vi "Estimate Ackermann Steering Frame.vi"(8 "error in (no error)":errorcluster, 11 "steering frame in":refnum<class "NI_Robotics_Steering Frame.lvclass">) -> (0 "error out":errorcluster, 2 "estimated ackermann steering frame copy":refnum<class "NI_Robotics_Ackermann Steering Frame.lvclass">, 3 "steering frame out":refnum<class "NI_Robotics_Steering Frame.lvclass">)   [LabVIEW 2017, in "NI_Robotics_Configure Steering Frame.lvlib"]
uses:
  <vilib>/robotics/Dialog/Configure Steering Frame/NI_Robotics_Configure Steering Frame.lvlib
  <vilib>/robotics/Steering/Steering Frame/NI_Robotics_Steering Frame.lvclass
  <vilib>/robotics/Steering/Ackermann Steering Frame/NI_Robotics_Ackermann Steering Frame.lvclass
  <vilib>/robotics/Steering/Steering Frame/NI_Robotics_Steering Frame.lvclass/NI_Robotics_Steering Frame.ctl
  <vilib>/robotics/Steering/Wheel/Wheel Parameters.ctl
  <vilib>/robotics/Steering/Wheel/Rotation Direction.ctl
  <vilib>/robotics/Steering/Steering Wheel/Steering Wheel Parameters.ctl
  <vilib>/robotics/Steering/Steering Wheel/Steering Angle Range.ctl
  <vilib>/robotics/Steering/Fixed Wheel/NI_Robotics_Fixed Wheel.lvclass
  c:/Program Files (x86)/National Instruments/LabVIEW 2017/vi.lib/robotics/Steering/Wheel/NI_Robotics_Wheel.lvclass
  <vilib>/robotics/Steering/Steering Wheel/NI_Robotics_Steering Wheel.lvclass
  <vilib>/robotics/Steering/Wheel/NI_Robotics_Wheel.lvclass/NI_Robotics_Wheel.ctl
  <vilib>/robotics/Steering/Steering Frame/Get Multiple Wheels in Steering Frame.vi
  <vilib>/robotics/Steering/Wheel/Get General Wheel Information.vi
  <vilib>/robotics/Steering/Wheel/Get Wheel Radius.vi
  <vilib>/robotics/Steering/Wheel/Get Motor Communication.vi
  <vilib>/robotics/Steering/Wheel/Get Wheel Parameters.vi
  <vilib>/robotics/Steering/Ackermann Steering Frame/Create Ackermann Steering Frame.vi
  <vilib>/robotics/Steering/Omnidirectional Wheel/Create Omnidirectional Wheel.vi
  <vilib>/robotics/Steering/Mecanum Wheel/Create Mecanum Wheel.vi
  <vilib>/robotics/Steering/Caster Wheel/Create Caster Wheel.vi
  <vilib>/robotics/Steering/Steering Wheel/Create Steering Wheel.vi
  <vilib>/robotics/Steering/Fixed Wheel/Create Fixed Wheel.vi
  <vilib>/robotics/Steering/Wheel/NI_Robotics_Wheel.lvclass
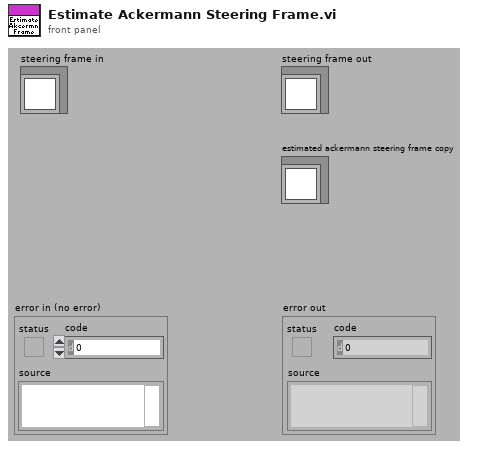
[diagram p1: front panel]
types:
  T1 = typedef "NI_Robotics_Steering Wheel.lvclass/Steering Wheel Parameters.ctl" = cluster{"steering gear ratio":dbl, "motor angle offset (rad)":dbl, "steering angle range":T2}
  T2 = typedef "NI_Robotics_Steering Wheel.lvclass/Steering Angle Range.ctl" = cluster{"min steering angle (rad)":dbl, "max steering angle (rad)":dbl}
  T3 = typedef "NI_Robotics_Wheel.lvclass/Wheel Parameters.ctl" = cluster{"wheel radius":dbl, "gear ratio":dbl, "forward rotation direction":T4}
  T4 = typedef "NI_Robotics_Wheel.lvclass/Rotation Direction.ctl" = u16
  T5 = cluster{"steering wheel out":refnum<class "NI_Robotics_Steering Wheel.lvclass">, "steering wheel out":refnum<class "NI_Robotics_Steering Wheel.lvclass">, "fixed wheel out":refnum<class "NI_Robotics_Fixed Wheel.lvclass">, "fixed wheel out":refnum<class "NI_Robotics_Fixed Wheel.lvclass">}
  T6 = cluster{"NI_Robotics_Steering Wheel.lvclass":refnum<class "NI_Robotics_Steering Wheel.lvclass">, "NI_Robotics_Steering Wheel.lvclass":refnum<class "NI_Robotics_Steering Wheel.lvclass">, "fixed wheel out":refnum<class "NI_Robotics_Fixed Wheel.lvclass">, "fixed wheel out":refnum<class "NI_Robotics_Fixed Wheel.lvclass">}
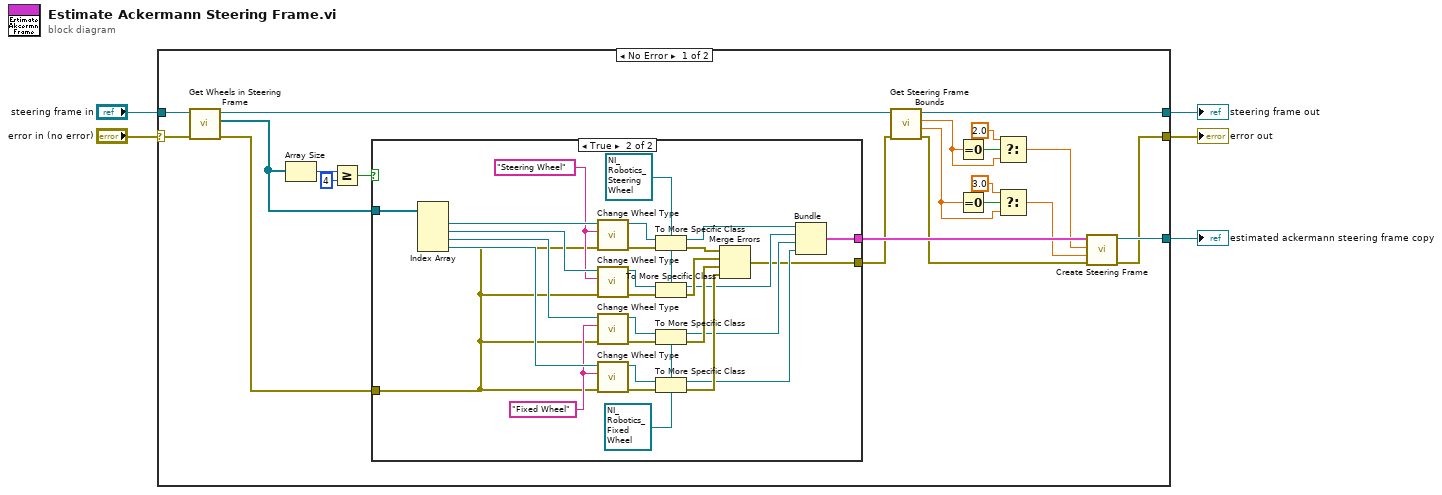
[diagram p0: block diagram]
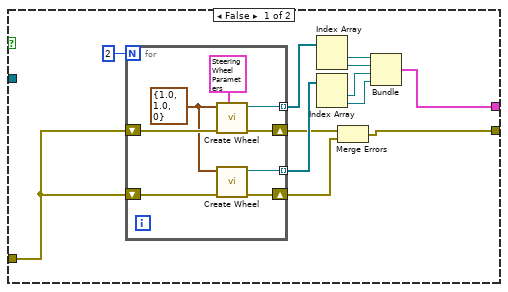
[diagram p2: hidden frame]
diagram:
  n1 = case shown="No Error" "error in (no error)" {
    selector: "error in (no error)" -> [w27 w77]
    tunnel: [w24 w77] -> w4
    tunnel: "steering frame in" -> [w26 w76]
    tunnel: [w11 w76] -> w2
    tunnel: [w25 _] -> w1
    frame No Error {
      n2 = call-poly <vilib>:"Get Wheels in Steering Frame.vi"("error in (no error)"=w27, "steering frame in"=w26) -> ("error out"=w19:errorcluster, "wheels"=w20:refnum<class "NI_Robotics_Wheel.lvclass">[], "steering frame out"=w6:refnum<class "NI_Robotics_Steering Frame.lvclass">)  [unwired: 3 in, 4 out]
      n3 = Array Size(array=w20) -> (size(s)=w23:i32)
      n4 = Greater Or Equal?(x=w23, y=4) -> (x >= y?=w21:bool)
      n5 = case shown="True" w21 {
        tunnel: w20 -> [_ w73]
        tunnel: w19 -> [w30 w48]
        tunnel: [w28 w50] -> w18
        tunnel: [w29 w49] -> w9
        frame False {
          n6 = for {
            N: 2 -> [_]
            shift-right: [w46] -> w33
            shift-left: w30 -> [w47]
            tunnel: [w45] -> w34 mode=indexing
            shift-right: [w43] -> w32
            shift-left: w30 -> [w44]
            tunnel: [w42] -> w35 mode=indexing
            w41 = T3 {"wheel radius"=1.0, "gear ratio"=1.0, "forward rotation direction"=0} ("wheel parameters")
            n7 = call-poly <vilib>:"Create Wheel.vi"("steering parameters"=T1 {"steering gear ratio"=1.0, "motor angle offset (rad)"=0.0, "steering angle range"={"min steering angle (rad)"=-3.14159, "max steering angle (rad)"=3.141592653589793}}, "error in (no error)"=w47, "wheel parameters"=w41) -> ("error out"=w46:errorcluster, "steering wheel out"=w45:refnum<class "NI_Robotics_Steering Wheel.lvclass">)  [unwired: 7 in]
            n8 = call-poly <vilib>:"Create Wheel.vi"("error in (no error)"=w44, "wheel parameters"=w41) -> ("error out"=w43:errorcluster, "fixed wheel out"=w42:refnum<class "NI_Robotics_Fixed Wheel.lvclass">)  [unwired: 8 in]
          }
          n9 = Index Array(array=w34) -> (element #1=w36:refnum<class "NI_Robotics_Steering Wheel.lvclass">, element #2=w37:refnum<class "NI_Robotics_Steering Wheel.lvclass">)  [unwired: 2 in]
          n10 = Index Array(array=w35) -> (element #1=w38:refnum<class "NI_Robotics_Fixed Wheel.lvclass">, element #2=w39:refnum<class "NI_Robotics_Fixed Wheel.lvclass">)  [unwired: 2 in]
          n11 = Merge Errors(w33, w32) -> (w29:errorcluster)
          n12 = Bundle("steering wheel out"=w36, "steering wheel out"=w37, "fixed wheel out"=w38, "fixed wheel out"=w39) -> (w28:T5)  [unwired: 1 in]
        }
        frame True {
          w61 = refnum<class "NI_Robotics_Steering Wheel.lvclass"> refnum ("NI_Robotics_Steering Wheel.lvclass")
          w64 = "Fixed Wheel" ("wheel type")
          w62 = refnum<class "NI_Robotics_Fixed Wheel.lvclass"> refnum ("fixed wheel out")
          w65 = "Steering Wheel" ("wheel type")
          n13 = Index Array(array=w73) -> (element #1=w72:refnum<class "NI_Robotics_Wheel.lvclass">, element #2=w68:refnum<class "NI_Robotics_Wheel.lvclass">, element #3=w67:refnum<class "NI_Robotics_Wheel.lvclass">, element #4=w66:refnum<class "NI_Robotics_Wheel.lvclass">)  [unwired: 4 in]
          n14 = call <vilib>:"Change Wheel Type.vi"("error in (no error)"=w48, "wheel type"=w65, "wheel in"=w72) -> ("error out"=w75:errorcluster, "wheel out"=w74:refnum<class "NI_Robotics_Wheel.lvclass">)  [unwired: 6 in, 1 out]
          n15 = call <vilib>:"Change Wheel Type.vi"("error in (no error)"=w48, "wheel type"=w65, "wheel in"=w68) -> ("error out"=w71:errorcluster, "wheel out"=w63:refnum<class "NI_Robotics_Wheel.lvclass">)  [unwired: 6 in, 1 out]
          n16 = call <vilib>:"Change Wheel Type.vi"("error in (no error)"=w48, "wheel type"=w64, "wheel in"=w67) -> ("error out"=w70:errorcluster, "wheel out"=w57:refnum<class "NI_Robotics_Wheel.lvclass">)  [unwired: 6 in, 1 out]
          n17 = call <vilib>:"Change Wheel Type.vi"("error in (no error)"=w48, "wheel type"=w64, "wheel in"=w66) -> ("error out"=w69:errorcluster, "wheel out"=w56:refnum<class "NI_Robotics_Wheel.lvclass">)  [unwired: 6 in, 1 out]
          n18 = To More Specific Class(target class=w61, reference=w74, error in=w75) -> (specific class reference=w54:refnum<class "NI_Robotics_Steering Wheel.lvclass">, error out=w60:errorcluster)
          n19 = To More Specific Class(target class=w61, reference=w63, error in=w71) -> (specific class reference=w53:refnum<class "NI_Robotics_Steering Wheel.lvclass">, error out=w59:errorcluster)
          n20 = To More Specific Class(target class=w62, reference=w57, error in=w70) -> (specific class reference=w52:refnum<class "NI_Robotics_Fixed Wheel.lvclass">, error out=w58:errorcluster)
          n21 = To More Specific Class(target class=w62, reference=w56, error in=w69) -> (specific class reference=w51:refnum<class "NI_Robotics_Fixed Wheel.lvclass">, error out=w55:errorcluster)
          n22 = Merge Errors(w60, w59, w58, w55) -> (w49:errorcluster)
          n23 = Bundle("NI_Robotics_Steering Wheel.lvclass"=w54, "NI_Robotics_Steering Wheel.lvclass"=w53, "fixed wheel out"=w52, "fixed wheel out"=w51) -> (w50:T6)  [unwired: 1 in]
        }
      }
      n24 = call <vilib>:"Get Steering Frame Bounds.vi"("error in (no error)"=w9, "steering frame in"=w6) -> ("error out"=w10:errorcluster, "length"=w17:dbl, "width"=w13:dbl, "steering frame out"=w11:refnum<class "NI_Robotics_Steering Frame.lvclass">)  [unwired: 4 in, 2 out]
      n25 = Equal To 0?(x=w13) -> (x = 0?=w12:bool)
      n26 = Equal To 0?(x=w17) -> (x = 0?=w15:bool)
      n27 = Select(t=2.0 ("wheel separation"), s=w12, f=w13) -> (s? t:f=w8:dbl)
      n28 = Select(t=3.0 ("wheel separation"), s=w15, f=w17) -> (s? t:f=w7:dbl)
      n29 = call-poly <vilib>:"Create Steering Frame.vi"("error in (no error)"=w10, "wheel separation length"=w7, "wheel separation width"=w8, "wheels"=w18) -> ("error out"=w24:errorcluster, "ackermann steering frame out"=w25:refnum<class "NI_Robotics_Ackermann Steering Frame.lvclass">)  [unwired: 6 in]
    }
    frame Error {
    }
  }
  "steering frame out" <- w2
  "error out" <- w4
  "estimated ackermann steering frame copy" <- w1
